vi "Move Picture.vi"(6 "Delta":cluster{"x":i16, "y":i16}, 8 "error in (no error)":errorcluster, 11 "Picture In":picture) -> (0 "error out":errorcluster, 3 "value":picture)   [LabVIEW 2023]
doc: "Wiebe Walstra\nwww.carya.nl"
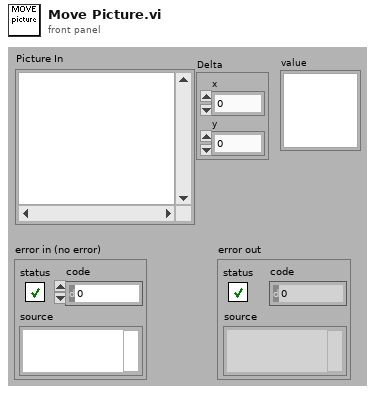
[diagram p1: front panel]
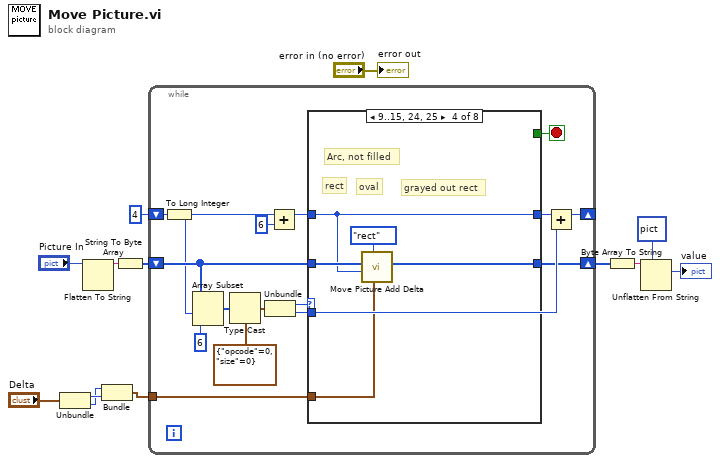
[diagram p0: block diagram]
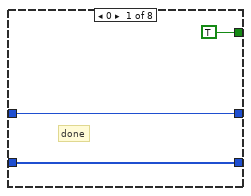
[diagram p2: hidden frame]
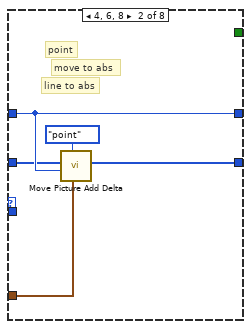
[diagram p3: hidden frame]
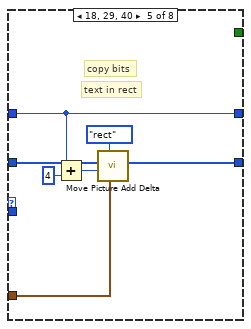
[diagram p5: hidden frame]
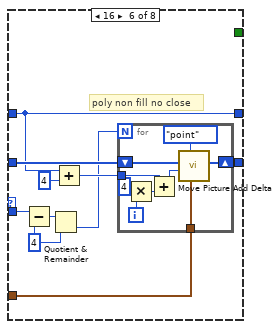
[diagram p6: hidden frame]
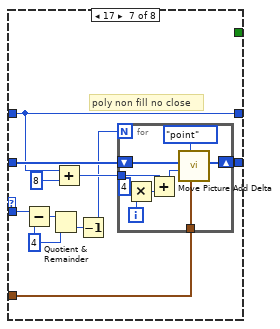
[diagram p7: hidden frame]
diagram:
  n1 = Unbundle("Delta") -> ("x"=w3:i16, "y"=w1:i16)
  n2 = Flatten To String(anything="Picture In") -> (data string=w13:string)  [unwired: 3 in, 2 out]
  n3 = Bundle("y"=w1, "x"=w3) -> (w2:cluster{"y":i16, "x":i16})  [unwired: 1 in]
  n4 = String To Byte Array(string=w13) -> (unsigned byte array=w11:u8[])
  n5 = while {
    shift-right: [w17] -> _
    shift-left: 4 -> [w25]
    shift-right: [w15] -> w7
    shift-left: w11 -> [w22]
    tunnel: w2 -> [w14]
    stop <- w23 stop-if-true
    n6 = To Long Integer(number=w25) -> (32bit integer=w20:i32)
    n7 = Array Subset(array=w22, index=w20, length=6 ("length (rest)")) -> (w24:u8[])
    n8 = Type Cast(type=cluster{"opcode":i16, "size":i32} {"opcode"=0, "size"=0}, x=w24) -> (*(type *) &x=w27:cluster{"opcode":i16, "size":i32})
    n9 = Unbundle(w27) -> ("opcode"=w26:i16, "size"=w18:i32)
    n10 = Add(x=w20, y=6) -> (x+y=w19:i32)
    n11 = case shown="9..15, 24, 25" w26 {
      tunnel: w22 -> [w30 w35 w38 w43 w50 w60 w80 w91]
      tunnel: w19 -> [w32 w37 w39 w41 w47 w59 w79 w92]
      tunnel: [w32 w37 w39 w41 w47 w59 w79 w92] -> w16
      tunnel: w18 -> [_ _ _ _ _ w61 w81 _]
      tunnel: [TRUE _ _ _ _ _ _ _] -> w23
      tunnel: [w30 w34 w38 w40 w46 w56 w75 w91] -> w15
      tunnel: w14 -> [_ w33 _ w42 w45 w52 w71 _]
      frame 0 {
        # "done"
      }
      frame 4, 6, 8 {
        # "line to abs"
        # "move to abs"
        # "point"
        n12 = call "Move Picture Add Delta.vi"("Delta"=w33, "Function"=enum16{"nop", "point", "rect"}."point", "index"=w37, "Picture In"=w35) -> ("Picture Out"=w34:u8[])  [unwired: 7 in]
      }
      frame 5, 7 {
        # "line to rel"
        # "move to rel"
      }
      frame 9..15, 24, 25 {
        # "Arc, not filled"
        # "grayed out rect"
        # "oval"
        # "rect"
        n13 = call "Move Picture Add Delta.vi"("Delta"=w42, "Function"=enum16{"nop", "point", "rect"}."rect", "index"=w41, "Picture In"=w43) -> ("Picture Out"=w40:u8[])  [unwired: 7 in]
      }
      frame 18, 29, 40 {
        # "copy bits"
        # "text in rect"
        n14 = Add(x=w47, y=4) -> (x+y=w48:i32)
        n15 = call "Move Picture Add Delta.vi"("Delta"=w45, "Function"=enum16{"nop", "point", "rect"}."rect", "index"=w48, "Picture In"=w50) -> ("Picture Out"=w46:u8[])  [unwired: 7 in]
      }
      frame 16 {
        w57 = 4 ("y")
        # "poly non fill no close"
        n16 = Subtract(x=w61, y=w57) -> (x-y=w58:i32)
        n17 = Quotient & Remainder(x=w58, y=w57) -> (floor(x/y)=w53:i32)  [unwired: 1 out]
        n18 = Add(x=w59, y=4) -> (x+y=w55:i32)
        n19 = for {
          N: w53 -> [_]
          tunnel: w55 -> [w63]
          shift-right: [w68] -> w56
          shift-left: w60 -> [w69]
          tunnel: w52 -> [w67]
          i -> [w66]
          n20 = Multiply(x=4, y=w66) -> (x*y=w64:i32)
          n21 = Add(x=w63, y=w64) -> (x+y=w62:i32)
          n22 = call "Move Picture Add Delta.vi"("Delta"=w67, "Function"=enum16{"nop", "point", "rect"}."point", "index"=w62, "Picture In"=w69) -> ("Picture Out"=w68:u8[])  [unwired: 7 in]
        }
      }
      frame 17 {
        w77 = 4 ("y")
        # "poly non fill no close"
        n23 = Subtract(x=w81, y=w77) -> (x-y=w78:i32)
        n24 = Quotient & Remainder(x=w78, y=w77) -> (floor(x/y)=w76:i32)  [unwired: 1 out]
        n25 = Add(x=w79, y=8) -> (x+y=w74:i32)
        n26 = Decrement(x=w76) -> (x-1=w72:i32)
        n27 = for {
          N: w72 -> [_]
          tunnel: w74 -> [w83]
          shift-right: [w88] -> w75
          shift-left: w80 -> [w89]
          tunnel: w71 -> [w87]
          i -> [w86]
          n28 = Multiply(x=4, y=w86) -> (x*y=w84:i32)
          n29 = Add(x=w83, y=w84) -> (x+y=w82:i32)
          n30 = call "Move Picture Add Delta.vi"("Delta"=w87, "Function"=enum16{"nop", "point", "rect"}."point", "index"=w82, "Picture In"=w89) -> ("Picture Out"=w88:u8[])  [unwired: 7 in]
        }
      }
      frame Default {
      }
    }
    n31 = Add(x=w16, y=w18) -> (x+y=w17:i32)
  }
  n32 = Byte Array To String(unsigned byte array=w7) -> (string=w6:string)
  n33 = Unflatten From String(type=picture data[5B] ("empty picture"), binary string=w6) -> (value=→"value":picture)  [unwired: 3 in, 2 out]
  "error out" <- "error in (no error)"
